vi "svx_Orbit Data Changed.vi"(0 "orbit plot X":dbl[](array[numeric]), 1 "shaft rotating direction":u16, 2 "probe angles X":dbl max=360.0 step=1.0, 3 "probe angles Y":dbl=90.0 max=360.0 step=1.0, 5 "orbit plot Y":dbl[](array[numeric]), 7 "actual samples/rev":dbl=64.0 format="%.2f", 9 "plot type":enum16{"Filtered Plot", "Unfiltered Plot"}(ring), 12 "trigger pulse direction":u16(ring)=1 items=["positive going", "negative going"]) -> (4 "orbit data":T1, 6 "tacho points":cluster{dbl[], dbl[]}, 8 "precession direction":u16[](array[ring]) items=["forward", "backward"], 10 "probe angles":cluster{"angles X":dbl, "angles Y":dbl}, 15 "elliptical info":cluster{"a":dbl, "b":dbl, "e":dbl, "ang":dbl}[](array[cluster]))   [LabVIEW 2017, in "SVX Orbit.xctl"]
uses:
  <vilib>/addons/_XControls/Orbit Plot/SVX Orbit.xctl
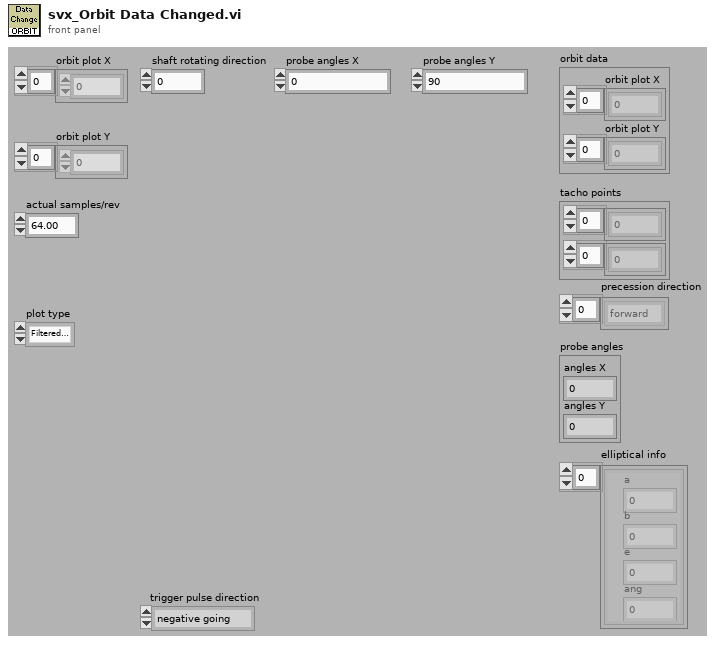
[diagram p1: front panel]
types:
  T1 = cluster{"orbit plot X":dbl[], "orbit plot Y":dbl[]}
  T2 = cluster{"probe angles X":dbl, "probe angles Y":dbl}
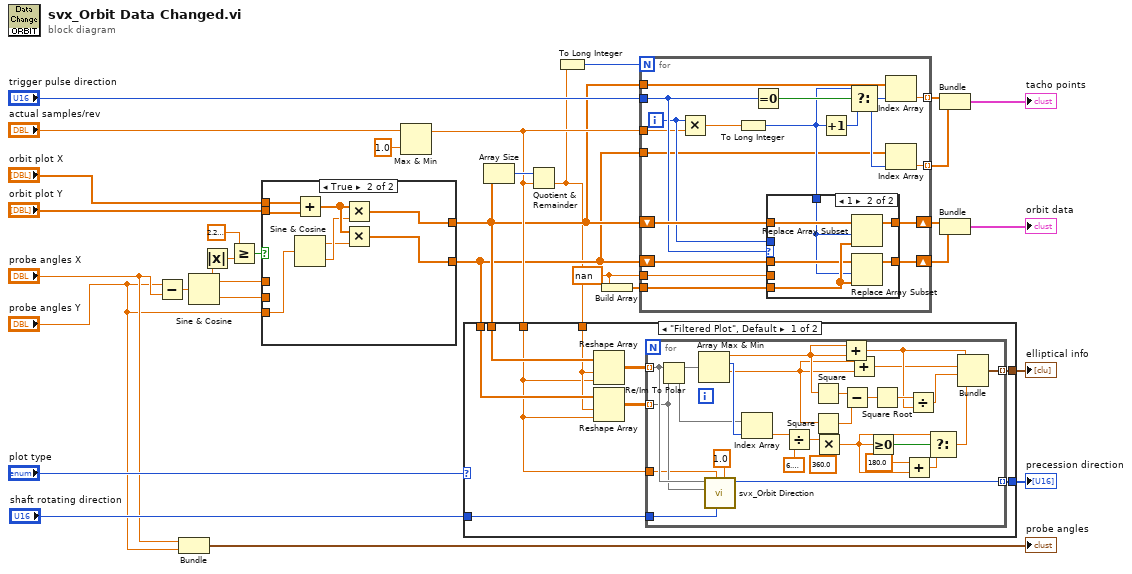
[diagram p0: block diagram]
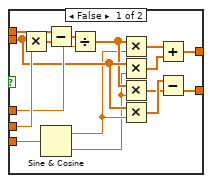
[diagram p3: hidden frame]
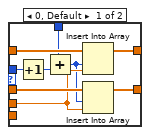
[diagram p4: hidden frame]
diagram:
  w26 = nan ("element")
  n1 = Subtract(x="probe angles Y", y="probe angles X") -> (x-y=w17:dbl)
  n2 = Bundle("probe angles X"="probe angles X", "probe angles Y"="probe angles Y") -> (→"probe angles":T2)  [unwired: 1 in]
  n3 = Sine & Cosine(0:w17) -> (1:w11:dbl, 2:w16:dbl)
  n4 = Absolute Value(x=w11) -> (abs(x)=w9:dbl)
  n5 = Greater Or Equal?(x=2.220446049250313e-16, y=w9) -> (x >= y?=w10:bool)
  n6 = case shown="True" w10 {
    tunnel: w16 -> [w48 _]
    tunnel: w11 -> [w46 _]
    tunnel: "probe angles Y" -> [w41 w53]
    tunnel: "orbit plot X" -> [w39 w56]
    tunnel: "orbit plot Y" -> [w42 w55]
    tunnel: [w34 w50] -> w7
    tunnel: [w33 w49] -> w6
    frame False {
      n7 = Multiply(x=w42, y=w48) -> (x*y=w45:dbl[])
      n8 = Sine & Cosine(0:w41) -> (1:w36:dbl, 2:w35:dbl)
      n9 = Subtract(x=w39, y=w45) -> (x-y=w47:dbl[])
      n10 = Divide(x=w47, y=w46) -> (x/y=w40:dbl[])
      n11 = Multiply(x=w40, y=w36) -> (x*y=w44:dbl[])
      n12 = Multiply(x=w42, y=w35) -> (x*y=w43:dbl[])
      n13 = Multiply(x=w40, y=w35) -> (x*y=w37:dbl[])
      n14 = Multiply(x=w42, y=w36) -> (x*y=w38:dbl[])
      n15 = Add(x=w44, y=w43) -> (x+y=w34:dbl[])
      n16 = Subtract(x=w38, y=w37) -> (x-y=w33:dbl[])
    }
    frame True {
      n17 = Add(x=w56, y=w55) -> (x+y=w54:dbl[])
      n18 = Sine & Cosine(0:w53) -> (1:w51:dbl, 2:w52:dbl)
      n19 = Multiply(x=w54, y=w52) -> (x*y=w50:dbl[])
      n20 = Multiply(x=w54, y=w51) -> (x*y=w49:dbl[])
    }
  }
  n21 = Max & Min(x="actual samples/rev", y=1.0) -> (max(x,y)=w13:dbl)  [unwired: 1 out]
  n22 = Array Size(array=w7) -> (size(s)=w24:i32)
  n23 = Quotient & Remainder(x=w24, y=w13) -> (floor(x/y)=w5:dbl)  [unwired: 1 out]
  n24 = case shown="\"Filtered Plot\", Default" "plot type" {
    tunnel: w7 -> [w65 _]
    tunnel: [w62 _] -> w14
    tunnel: w6 -> [w61 _]
    tunnel: w13 -> [w59 _]
    tunnel: w5 -> [w60 _]
    tunnel: "shaft rotating direction" -> [w58 _]
    tunnel: [w57 _] -> w3
    frame "Filtered Plot", Default {
      n25 = Reshape Array(w65, w60, w59) -> (w64:dbl[][])
      n26 = Reshape Array(w61, w60, w59) -> (w63:dbl[][])
      n27 = for {
        tunnel: w64 -> [w71] mode=indexing
        tunnel: w63 -> [w70] mode=indexing
        tunnel: [w76] -> w62 mode=indexing
        tunnel: w59 -> [w69]
        tunnel: w58 -> [w67]
        tunnel: [w66] -> w57 mode=indexing
        n28 = Re/Im To Polar(2:w70, 3:w71) -> (0:w84:dbl[], 1:w93:dbl[])
        n29 = Array Max & Min(array=w93) -> (max value=w75:dbl, max index (indices)=w85:i32, min value=w73:dbl)  [unwired: 1 out]
        n30 = call <vilib>:"svx_Orbit Direction.vi"("revolutions"=1.0, "shaft rotating direction"=w67, "actual samples/rev"=w69, "orbit plot Y"=w70, "orbit plot X"=w71) -> ("orbit precession direction"=w66:u16)  [unwired: 6 in]
        n31 = Index Array(array=w84, index=w85) -> (element=w83:dbl)
        n32 = Divide(x=w83, y=6.283185307179586) -> (x/y=w91:dbl)
        n33 = Square(x=w75) -> (x^2=w81:dbl)
        n34 = Square(x=w73) -> (x^2=w82:dbl)
        n35 = Multiply(x=w91, y=360.0) -> (x*y=w89:dbl)
        n36 = Add(x=w75, y=w75) -> (x+y=w74:dbl)
        n37 = Subtract(x=w81, y=w82) -> (x-y=w80:dbl)
        n38 = Add(x=w73, y=w73) -> (x+y=w72:dbl)
        n39 = Greater Or Equal To 0?(x=w89) -> (x >= 0?=w87:bool)
        n40 = Square Root(x=w80) -> (sqrt(x)=w79:dbl)
        n41 = Add(x=180.0, y=w89) -> (x+y=w86:dbl)
        n42 = Divide(x=w79, y=w74) -> (x/y=w78:dbl)
        n43 = Select(t=w89, s=w87, f=w86) -> (s? t:f=w77:dbl)
        n44 = Bundle(w74, w72, w78, w77) -> (w76:cluster{dbl, dbl, dbl, dbl})  [unwired: 1 in]
      }
    }
    frame "Unfiltered Plot" {
    }
  }
  "elliptical info" <- w14
  "precession direction" <- w3
  n45 = To Long Integer(number=w5) -> (32bit integer=w30:i32)
  n46 = Build Array(w26) -> (w25:dbl[])
  n47 = for {
    N: w30 -> [_]
    tunnel: w13 -> [w94]
    tunnel: "trigger pulse direction" -> [w103]
    tunnel: [w111] -> w32 mode=indexing
    tunnel: [w110] -> w31 mode=indexing
    tunnel: w25 -> [w107]
    shift-right: [w105] -> w29
    shift-left: w7 -> [w106]
    shift-right: [w104] -> w28
    shift-left: w6 -> [w100]
    tunnel: w26 -> [w102]
    tunnel: w7 -> [w97]
    tunnel: w6 -> [w96]
    i -> [w101]
    n48 = Multiply(x=w101, y=w94) -> (x*y=w95:dbl)
    n49 = To Long Integer(number=w95) -> (32bit integer=w99:i32)
    n50 = Equal To 0?(x=w103) -> (x = 0?=w109:bool)
    n51 = case shown="1" w103 {
      tunnel: w107 -> [_ w126]
      tunnel: w106 -> [w120 w125]
      tunnel: [w113 w124] -> w105
      tunnel: w100 -> [w119 w123]
      tunnel: [w112 w122] -> w104
      tunnel: w99 -> [w117 w121]
      tunnel: w102 -> [w118 _]
      tunnel: w101 -> [w116 _]
      frame 0, Default {
        n52 = Increment(x=w116) -> (x+1=w114:i32)
        n53 = Add(x=w117, y=w114) -> (x+y=w115:i32)
        n54 = Insert Into Array(array=w120, index=w115, new element=w118) -> (w113:dbl[])
        n55 = Insert Into Array(array=w119, index=w115, new element=w118) -> (w112:dbl[])
      }
      frame 1 {
        n56 = Replace Array Subset(array=w125, new element=w126, index=w121) -> (w124:dbl[])
        n57 = Replace Array Subset(array=w123, new element=w126, index=w121) -> (w122:dbl[])
      }
    }
    n58 = Increment(x=w99) -> (x+1=w98:i32)
    n59 = Select(t=w99, s=w109, f=w98) -> (s? t:f=w108:i32)
    n60 = Index Array(array=w97, index=w108) -> (element=w111:dbl)
    n61 = Index Array(array=w96, index=w108) -> (element=w110:dbl)
  }
  n62 = Bundle(w32, w31) -> (→"tacho points":cluster{dbl[], dbl[]})  [unwired: 1 in]
  n63 = Bundle(w29, w28) -> (→"orbit data":cluster{dbl[], dbl[]})  [unwired: 1 in]
